vi "StartNewPanel.vi"() -> ()   [LabVIEW 2015]
uses:
  GlobalData.vi
  GlobalPath.vi
  GlobalVi.vi
panel:
  out "Panel Type":string
  out "Log File extension":string
  in  "Create log file?":bool
  in  "Done ?":bool
  in  "String 2":string
  in  "String":string
  in  "Open DB":bool
  in  "Done with adding new panel?":bool
  # "Adding a new panel in the database"
  # "Add>Add then from the list choose \"Readout\" and then Start\nChoose the correct ID and click \"Start building panel\""
  # "(Leave the database window open in the background)"
  # "Creating a log file"
  # "R"
  # "S1-0000-00"
  # "(in the first field add \"S\" for stereo and \"E\" for eta panel e.g. RSE1-0000-0005)"
  # "Panel name:"
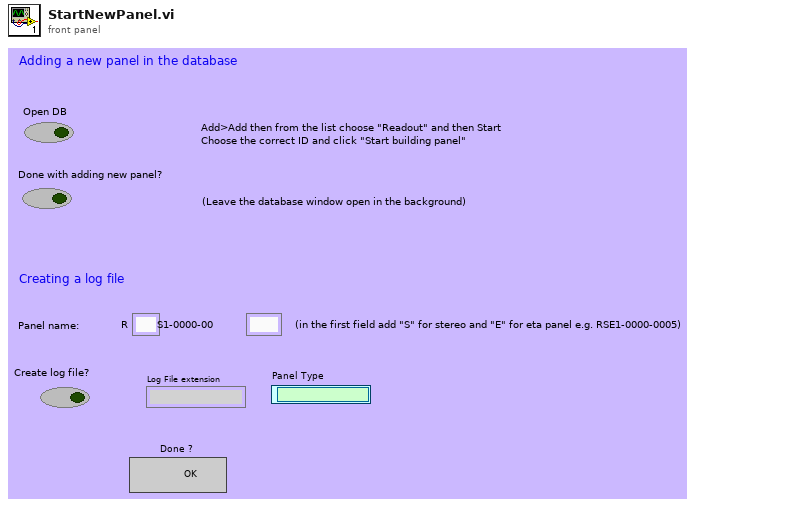
[diagram p1: front panel]
types:
  T1 = enum16{"open", "replace", "create", "open or create", "replace or create", "replace or create with confirmation"}
  T2 = enum32{"Bad", "Idle", "Run top level", "Running"}
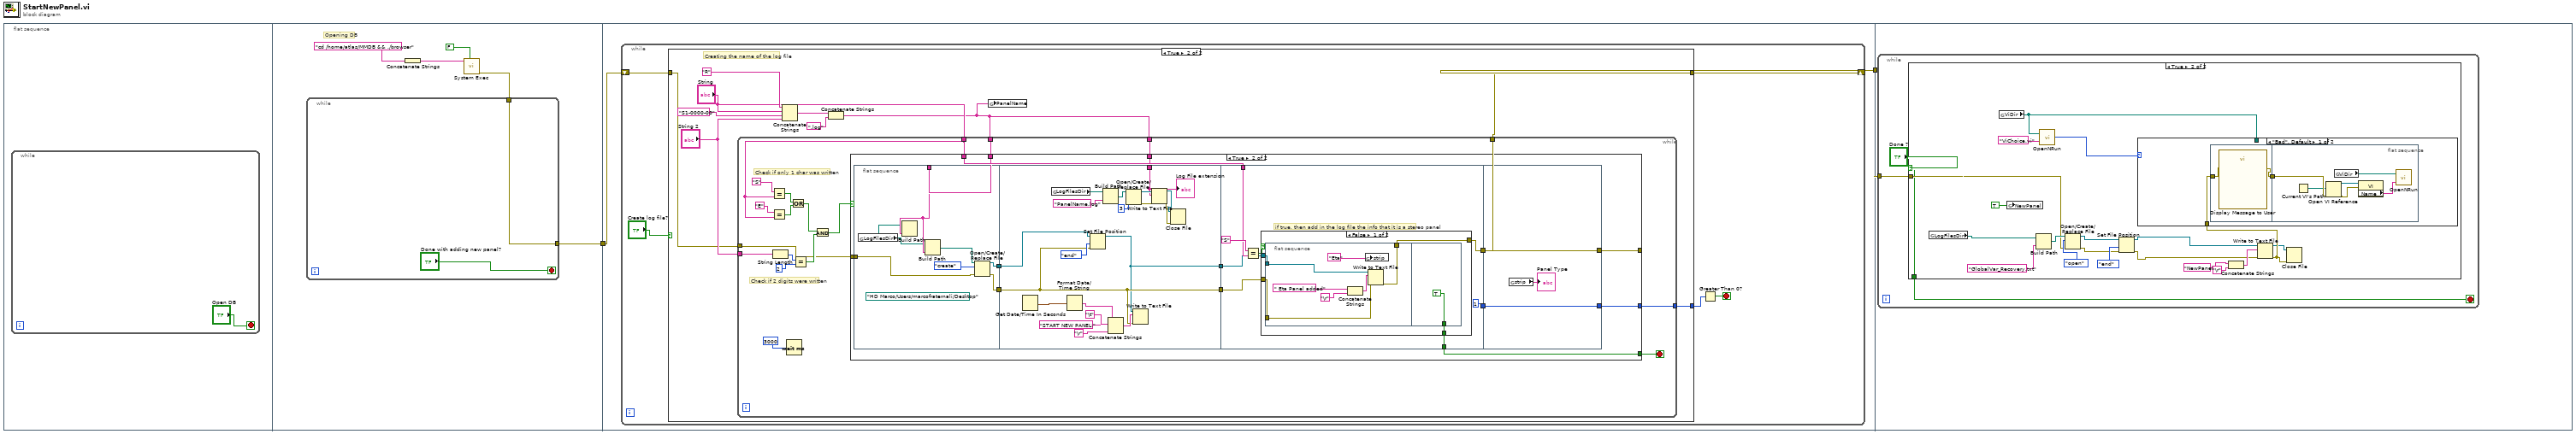
[diagram p0: block diagram]
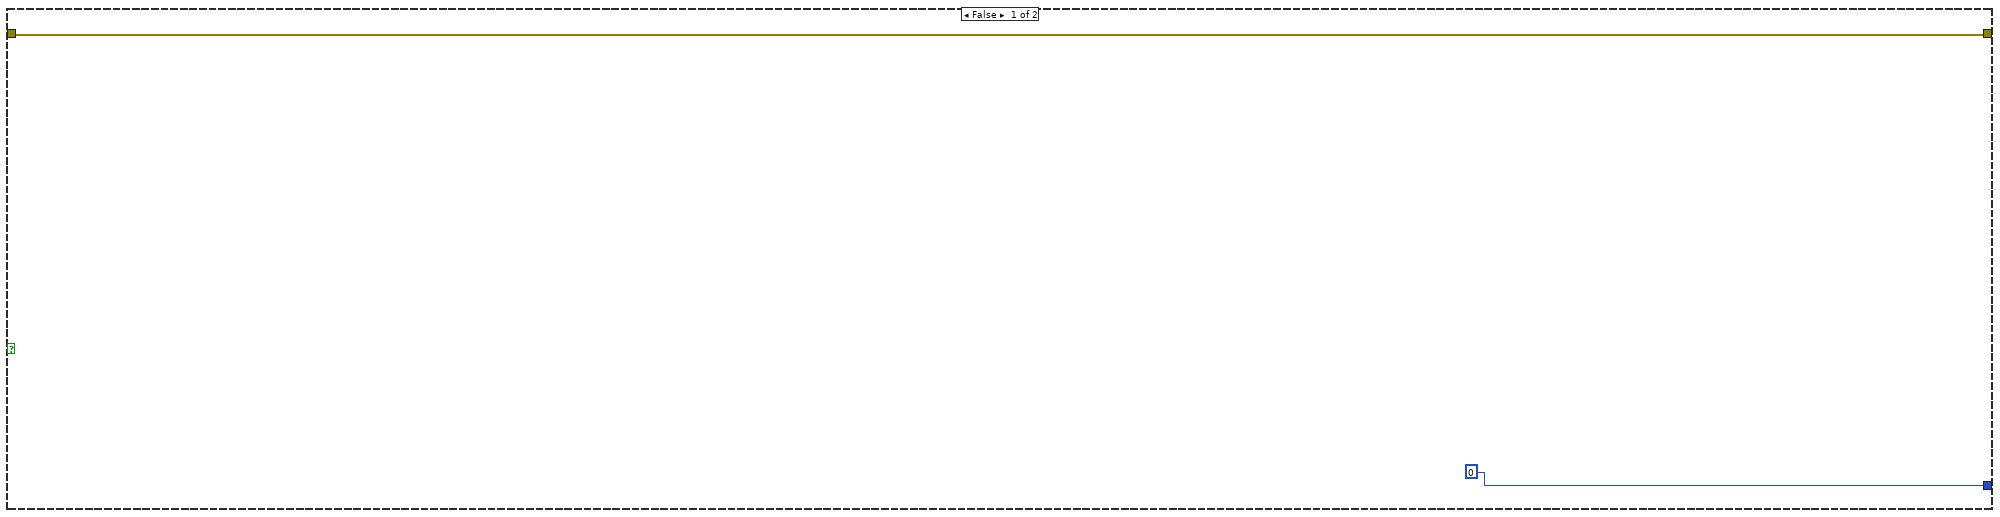
[diagram p2: hidden frame]
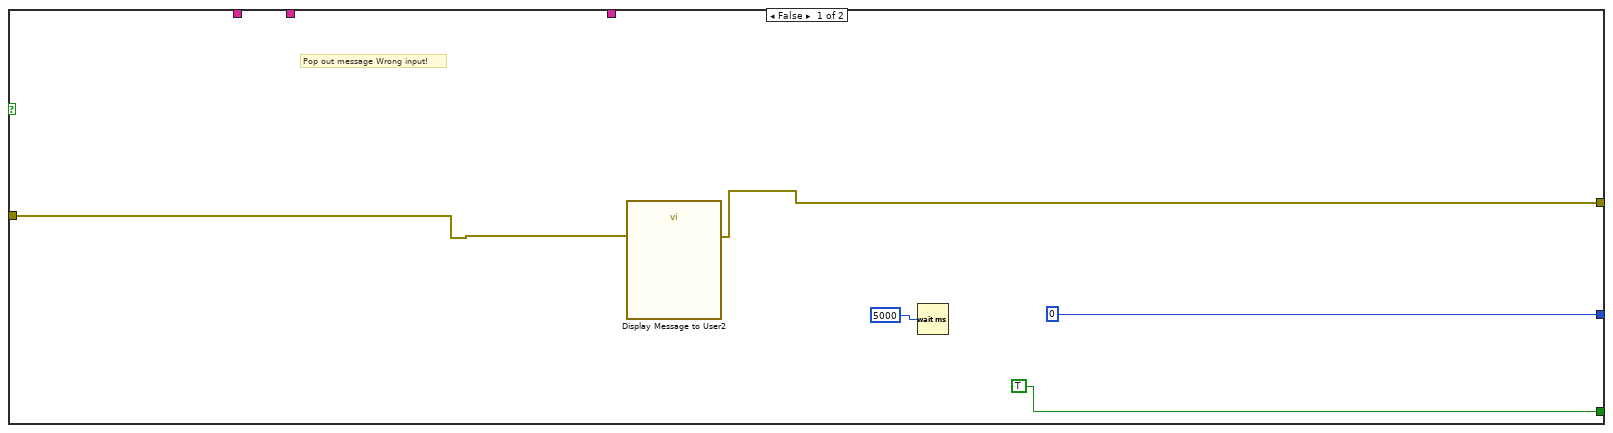
[diagram p3: hidden frame]
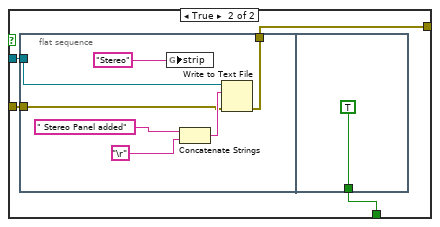
[diagram p4: hidden frame]
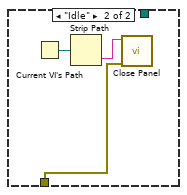
[diagram p6: hidden frame]
diagram:
  n1 = flat-sequence {
    tunnel: [w8] -> w2
    tunnel: w2 -> [w12]
    tunnel: [w11] -> w1
    tunnel: w1 -> [w127]
    frame #0 {
      n2 = while {
        stop <- "Open DB" stop-if-true
      }
    }
    frame #1 {
      # "Opening DB"
      n3 = Concatenate Strings("cd /home/atlas/MMDB && ./browser") -> (w6:string)
      n4 = call <vilib>:"System Exec.vi"("wait until completion? (T)"=FALSE, "command line"=w6) -> ("error out"=w5:errorcluster)  [unwired: 6 in, 3 out]
      n5 = while {
        tunnel: [w9] -> w8
        tunnel: w5 -> [w9]
        stop <- "Done with adding new panel?" stop-if-true
      }
    }
    frame #2 {
      n6 = while {
        shift-right: [w13] -> w11
        shift-left: w12 -> [w17]
        stop <- w16 stop-if-true
        n7 = case shown="True" "Create log file?" {
          tunnel: w17 -> [w18 w24]
          tunnel: [0 w23] -> w15
          tunnel: [w18 w22] -> w13
          frame False {
          }
          frame True {
            # "Creating the name of the log file"
            n8 = Concatenate Strings("R", "String", "S1-0000-00", "String 2") -> (w21:string)
            n9 = Concatenate Strings(w21, ".log") -> (w20:string)
            n10 = while {
              tunnel: "String" -> [w46]
              tunnel: w20 -> [w42]
              tunnel: "String 2" -> [w40]
              tunnel: w24 -> [w34]
              tunnel: [w33] -> w22
              tunnel: [w32] -> w23
              tunnel: w20 -> [w30]
              stop <- w41 stop-if-true
              # "Check if 2 digits were written"
              # "Check if only 1 char was written"
              n11 = Equal?(x="S", y=w46) -> (x = y?=w44:bool)
              n12 = Equal?(x="E", y=w46) -> (x = y?=w43:bool)
              n13 = String Length(string=w40) -> (length=w39:i32)
              n14 = Wait (ms)(milliseconds to wait=3000) -> ()  [unwired: 1 out]
              n15 = Or(x=w44, y=w43) -> (x .or. y?=w36:bool)
              n16 = Equal?(x=w39, y=2) -> (x = y?=w37:bool)
              n17 = And(x=w36, y=w37) -> (x .and. y?=w35:bool)
              n18 = case shown="True" w35 {
                tunnel: w46 -> [_ w65]
                tunnel: w42 -> [_ w56]
                tunnel: [TRUE w64] -> w41
                tunnel: w34 -> [w51 w63]
                tunnel: [w50 w62] -> w33
                tunnel: [0 w57] -> w32
                tunnel: w30 -> [_ w55]
                frame False {
                  # "Pop out message Wrong input!"
                  n19 = call "Display Message to User2"("error in (no error)"=w51) -> ("error out"=w50:errorcluster)  [unwired: 9 in, 1 out]
                  n20 = Wait (ms)(milliseconds to wait=5000) -> ()  [unwired: 1 out]
                }
                frame True {
                  n21 = flat-sequence {
                    tunnel: w56 -> [w67]
                    tunnel: [w68] -> w61
                    tunnel: w63 -> [w71]
                    tunnel: [w70] -> w59
                    tunnel: w61 -> [w84]
                    tunnel: [w83] -> w60
                    tunnel: w59 -> [w85]
                    tunnel: [w85] -> w58
                    tunnel: w55 -> [w75]
                    tunnel: w65 -> [w97]
                    tunnel: w60 -> [w96]
                    tunnel: [w95] -> w64
                    tunnel: w58 -> [w94]
                    tunnel: [w93] -> w54
                    tunnel: [1] -> w53
                    tunnel: [w125] -> w57
                    tunnel: [w126] -> w62
                    tunnel: w54 -> [w126]
                    tunnel: w53 -> [w125]
                    frame #0 {
                      (unwired) path "/HD Marco/Users/marcofraternali/Desktop" ("path")
                      n22 = global read "GlobalPath.vi" "LogFilesDir"() -> (w66:path)
                      n23 = Build Path(base path=w66, name or relative path=w67) -> ()  [unwired: 1 out]
                      n24 = Build Path(base path=w66, name or relative path=w67) -> (appended path=w72:path)
                      n25 = Open/Create/Replace File(file path (use dialog)=w72, error in=w71, operation (0:open)=T1."create") -> (refnum out=w68:refnum<file>, error out=w70:errorcluster)  [unwired: 3 in, 1 out]
                    }
                    frame #1 {
                      n26 = Get Date/Time In Seconds() -> (seconds since 1Jan1904=w82:timestamp)
                      n27 = global read "GlobalPath.vi" "LogFilesDir"() -> (w76:path)
                      n28 = Format Date/Time String(seconds (now)=w82) -> (date/time string=w89:string)  [unwired: 2 in]
                      n29 = Set File Position(refnum=w84, from (0:start)=enum16{"start", "end", "current"}."end", error in=w85) -> (refnum out=w83:refnum<file>)  [unwired: 1 in, 1 out]
                      n30 = Build Path(base path=w76, name or relative path="PanelName.log") -> (appended path=w78:path)
                      n31 = Concatenate Strings(w89, "\t", "START NEW PANEL:", "\r") -> (w87:string)
                      n32 = Open/Create/Replace File(file path (use dialog)=w78, operation (0:open)=3) -> (refnum out=w81:refnum<file>, error out=w80:errorcluster)  [unwired: 4 in, 1 out]
                      n33 = Write to Text File(file (use dialog)=w83, text=w87, error in=w85) -> ()  [unwired: 1 in, 3 out]
                      n34 = Write to Text File(file (use dialog)=w81, text=w75, error in=w80) -> (refnum out=w74:refnum<file>, error out=w73:errorcluster)  [unwired: 1 in, 1 out]
                      n35 = Close File(refnum=w74, error in=w73) -> ()  [unwired: 2 out]
                      "Log File extension" <- w75
                    }
                    frame #2 {
                      # "if true, then add in the log file the info that it is a stereo panel"
                      n36 = Equal?(x="S", y=w97) -> (x = y?=w99:bool)
                      n37 = case shown="False" w99 {
                        tunnel: w96 -> [w103 w115]
                        tunnel: [w102 w114] -> w95
                        tunnel: w94 -> [w101 w113]
                        tunnel: [w100 w112] -> w93
                        frame False {
                          n38 = flat-sequence {
                            tunnel: w103 -> [w110]
                            tunnel: w101 -> [w107]
                            tunnel: [w106] -> w100
                            tunnel: [TRUE] -> w102
                            frame #0 {
                              n39 = Concatenate Strings(" Eta Panel added", "\r") -> (w109:string)
                              n40 = global write "GlobalData.vi" "strip"("Eta") -> ()
                              n41 = Write to Text File(file (use dialog)=w110, text=w109, error in=w107) -> (error out=w106:errorcluster)  [unwired: 1 in, 2 out]
                            }
                            frame #1 {
                            }
                          }
                        }
                        frame True {
                          n42 = flat-sequence {
                            tunnel: w115 -> [w122]
                            tunnel: w113 -> [w119]
                            tunnel: [w118] -> w112
                            tunnel: [TRUE] -> w114
                            frame #0 {
                              n43 = global write "GlobalData.vi" "strip"("Stereo") -> ()
                              n44 = Concatenate Strings(" Stereo Panel added", "\r") -> (w121:string)
                              n45 = Write to Text File(file (use dialog)=w122, text=w121, error in=w119) -> (error out=w118:errorcluster)  [unwired: 1 in, 2 out]
                            }
                            frame #1 {
                            }
                          }
                        }
                      }
                    }
                    frame #3 {
                      n46 = global read "GlobalData.vi" "strip"() -> (→"Panel Type":string)
                    }
                  }
                }
              }
            }
            n47 = global write "GlobalData.vi" "PanelName"(w20) -> ()
          }
        }
        n48 = Greater Than 0?(x=w15) -> (x > 0?=w16:bool)
      }
    }
    frame #3 {
      n49 = while {
        tunnel: w127 -> [w130]
        stop <- w128 stop-if-true
        n50 = case shown="True" "Done ?" {
          selector: "Done ?" -> [w131 w148]
          tunnel: w130 -> [_ w140]
          tunnel: [w131 w148] -> w128
          frame False {
          }
          frame True {
            n51 = global read "GlobalPath.vi" "LogFilesDir"() -> (w134:path)
            n52 = global read "GlobalPath.vi" "ViDir"() -> (w149:path)
            n53 = global write "GlobalVi.vi" "NewPanel"(TRUE) -> ()
            n54 = Build Path(base path=w134, name or relative path="GlobalVar_Recovery.txt") -> (appended path=w145:path)
            n55 = call "OpenNRun.vi"("VI name"="ViChoice.vi", "ViDirPath"=w149) -> ("Execution:State"=w151:T2)
            n56 = Open/Create/Replace File(file path (use dialog)=w145, error in=w140, operation (0:open)=T1."open") -> (refnum out=w141:refnum<file>, error out=w142:errorcluster)  [unwired: 3 in, 1 out]
            n57 = Set File Position(refnum=w141, from (0:start)=enum16{"start", "end", "current"}."end", error in=w142) -> (refnum out=w137:refnum<file>, error out=w136:errorcluster)  [unwired: 1 in]
            n58 = Concatenate Strings("NewPanel", "\r") -> (w139:string)
            n59 = Write to Text File(file (use dialog)=w137, text=w139, error in=w136) -> (refnum out=w132:refnum<file>, error out=w133:errorcluster)  [unwired: 1 in, 1 out]
            n60 = case shown="\"Bad\", Default" w151 {
              tunnel: w149 -> [_ _]
              tunnel: w133 -> [w152 w162]
              frame "Bad", Default {
                n61 = flat-sequence {
                  tunnel: w152 -> [w155]
                  tunnel: [w154] -> w153
                  tunnel: w153 -> [w158]
                  frame #0 {
                    n62 = call "Display Message to User"("error in (no error)"=w155) -> ("error out"=w154:errorcluster)  [unwired: 9 in, 1 out]
                  }
                  frame #1 {
                    n63 = Current VI's Path() -> (path=w156:path)
                    n64 = Open VI Reference(vi path=w156, error in (no error)=w158) -> (vi reference=w161:refnum<vi>, error out=w160:errorcluster)  [unwired: 4 in]
                    n65 = global read "GlobalPath.vi" "ViDir"() -> (w157:path)
                    n66 = property class="VI"(reference=w161, error in=w160) -> ("Name"=w159:string)  [unwired: 2 out]
                    n67 = call "OpenNRun.vi"("VI name"=w159, "ViDirPath"=w157) -> ()  [unwired: 1 out]
                  }
                }
              }
              frame "Idle" {
                n68 = Current VI's Path() -> (path=w163:path)
                n69 = Strip Path(path=w163) -> (name=w164:string)  [unwired: 1 out]
                n70 = call <vilib>:"Close Panel.vi"("error in (no error)"=w162, "VI name"=w164) -> ()  [unwired: 9 in, 1 out]
              }
            }
            n71 = Close File(refnum=w132, error in=w133) -> ()  [unwired: 2 out]
          }
        }
      }
    }
  }
